vi "Read Stored Waveform Burst Length.vi"(0 "Instrument Handle in":refnum<k15>, 5 "Waveform Name":string, 11 "error in":errorcluster) -> (4 "Instrument Handle out":refnum<k15>, 6 "Waveform Burst Length (s)":dbl, 15 "error out":errorcluster)   [LabVIEW 2018, in "RDLUtilities.lvlib"]
uses:
  RDLUtilities.lvlib
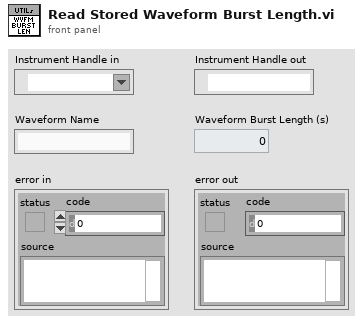
[diagram p1: front panel]
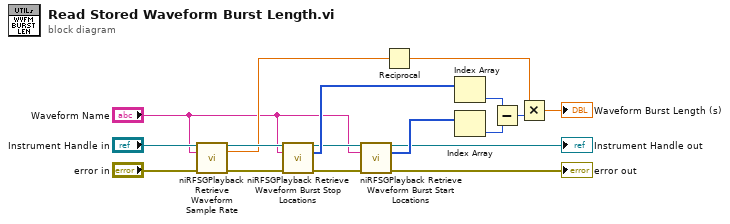
[diagram p0: block diagram]
diagram:
  n1 = call <instrlib>:"niRFSGPlayback Retrieve Waveform Sample Rate.vi"("instrument handle in"="Instrument Handle in", "waveform name"="Waveform Name", "error in"="error in") -> ("instrument handle out"=w12:refnum<k15>, "sample rate"=w8:dbl, "error out"=w11:errorcluster)  [unwired: 10 in]
  n2 = call <instrlib>:"niRFSGPlayback Retrieve Waveform Burst Stop Locations.vi"("instrument handle in"=w12, "waveform name"="Waveform Name", "error in"=w11) -> ("instrument handle out"=w10:refnum<k15>, "burst stop locations"=w17:i32[], "error out"=w13:errorcluster)  [unwired: 10 in]
  n3 = call <instrlib>:"niRFSGPlayback Retrieve Waveform Burst Start Locations.vi"("instrument handle in"=w10, "waveform name"="Waveform Name", "error in"=w13) -> ("instrument handle out"=→"Instrument Handle out":refnum<k15>, "burst start locations"=w16:i32[], "error out"=→"error out":errorcluster)  [unwired: 10 in]
  n4 = Reciprocal(x=w8) -> (1/x=w6:dbl)
  n5 = Index Array(array=w17) -> (element=w15:i32)  [unwired: 1 in]
  n6 = Index Array(array=w16) -> (element=w14:i32)  [unwired: 1 in]
  n7 = Subtract(x=w15, y=w14) -> (x-y=w9:i32)
  n8 = Multiply(x=w6, y=w9) -> (x*y=→"Waveform Burst Length (s)":dbl)
